vi "Auto Match.vi"() -> ()   [LabVIEW 2014]
panel:
  in  "stop":bool
  out "# of iterations":i32
  out "Currnet Number":dbl format="%#.0f"
  in  "Number to Match":dbl=50.0 min=0.0 max=1000.0 step=1.0 format="%#.0f"
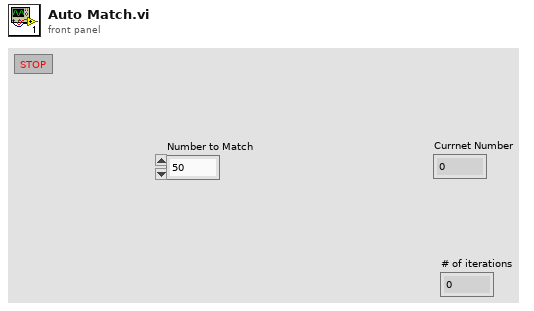
[diagram p1: front panel]
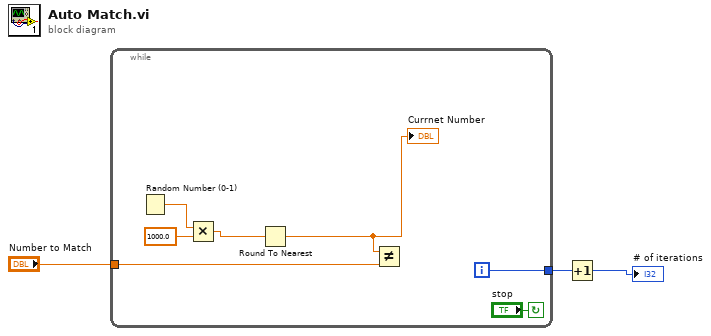
[diagram p0: block diagram]
diagram:
  n1 = while {
    tunnel: "Number to Match" -> [w5]
    tunnel: [w4] -> w1
    i -> [w4]
    stop <- "stop" continue-if-true
    n2 = Random Number (0-1)() -> (number: 0 to 1=w10:dbl)
    n3 = Multiply(x=w10, y=1000.0) -> (x*y=w8:dbl)
    n4 = Round To Nearest(number=w8) -> (nearest integer value=w7:dbl)
    "Currnet Number" <- w7
    n5 = Not Equal?(x=w7, y=w5) -> ()  [unwired: 1 out]
  }
  n6 = Increment(x=w1) -> (x+1=→"# of iterations":i32)
